vi "Pack Data and Write to Inline.vi"(8 "Error In":errorcluster, 10 "Injection Event Data Cluster":T1 {"Shots"."Results"."Off-Stage Avg Current" format="%#.6g"; "Shots"."Results"."Total Voltage Pulses" format="%#.6g"; "Shots"."Results"."Off-Stage Min Current" format="%#.6g"; "Shots"."Results"."Off-Stage Max Current" format="%#.6g"}, 11 "Async Parameters":T4={"Name"="", "Rate.Hz"=0, "Injectors.Count"=0, "Injector.Timeout"=0.0, "Injector.Timer"=[], "Injector.Info"=[], "Events.Count"=[], "Event.Parameters"={"Shots"=0, "Shot.InitialVoltage"=0.0, "Shot.Stages"=0, "Stages"=[{"Stage.Dwell.Level"=0.0, "PullIn.Type"=enum."Pull In Transition Dwells", "PullIn.Level"=0.0, "Transition.Type"=enum."Stage Transition Voltage Level", "Transition.Level"=0.0}]}, "DMA.Ref"=refnum, "Waveform.Refs"=[], "Waveform.Sessions"=[], "Waveform.Enable"=refnum, "FPGA.Status"=refnum, "Search.Data"=refnum, "Results.Data"=refnum, "Results.Values"=[], "Results.Selections"=[]}) -> (0 "Error out":errorcluster, 3 "Async Parameters out":T4={"Name"="", "Rate.Hz"=0, "Injectors.Count"=0, "Injector.Timeout"=0.0, "Injector.Timer"=[], "Injector.Info"=[], "Events.Count"=[], "Event.Parameters"={"Shots"=0, "Shot.InitialVoltage"=0.0, "Shot.Stages"=0, "Stages"=[{"Stage.Dwell.Level"=0.0, "PullIn.Type"=enum."Pull In Transition Dwells", "PullIn.Level"=0.0, "Transition.Type"=enum."Stage Transition Voltage Level", "Transition.Level"=0.0}]}, "DMA.Ref"=refnum, "Waveform.Refs"=[], "Waveform.Sessions"=[], "Waveform.Enable"=refnum, "FPGA.Status"=refnum, "Search.Data"=refnum, "Results.Data"=refnum, "Results.Values"=[], "Results.Selections"=[]})   [LabVIEW 2015, in "Fuel Injection Addon Engine.lvlib"]
uses:
  Fuel Injection Addon Engine.lvlib
  Types/Async Parameters.ctl
  Shared/Types/Injector info.ctl
  Shared/Types/Shot.Parameters.ctl
  Shared/Types/Stage.Parameters.ctl
  Shared/Types/Stage.PullIn.Types.ctl
  Shared/Types/Stage.Transition.Types.ctl
  <vilib>/NI Veristand/Custom Device API/Waveform Data Reference.ctl
  <vilib>/NI VeriStand/Custom Device Waveform API/Single Waveform Write (DBL)/Single Waveform Write (DBL).lvclass
  <vilib>/NI/NIVS Inline Async API/_Data Access Engine/Data Access Engine/Types/Read.DVR.ctl
  <vilib>/NI/NIVS Inline Async API/_Data Access Engine/Access Type Classes/Read/Read.lvclass
  <vilib>/NI/NIVS Inline Async API/_Data Access Engine/Data Access Engine/Types/Write.DVR.ctl
  <vilib>/NI/NIVS Inline Async API/_Data Access Engine/Access Type Classes/Write/Write.lvclass
  Shared/Types/Analysis.Channels.Select.ctl
  Types/Injector Event Data Cluster.ctl
  RT Analysis/Controls/Shot Information Control.ctl
  Types/Boost Stage Current Measurements Cluster Control.ctl
  <vilib>/NI/NIVS Inline Async API/_Data Access Engine/Access Type Classes/Write/Write.lvclass/Write.ctl
  <vilib>/NI/NIVS Inline Async API/_Data Access Engine/Data Access Engine/Methods/Write.Data.vi
  <vilib>/NI/NIVS Inline Async API/_Data Access Engine/Access Type Classes/Write/Write.ProcessData.vi
  <vilib>/NI/NIVS Inline Async API/_Data Access Engine/Data Access Engine/Data Access Engine.lvclass
  Shared/Fuel Injection Addon Shared.lvlib
  <vilib>/NI VeriStand/Custom Device API/Custom Device API.lvlib
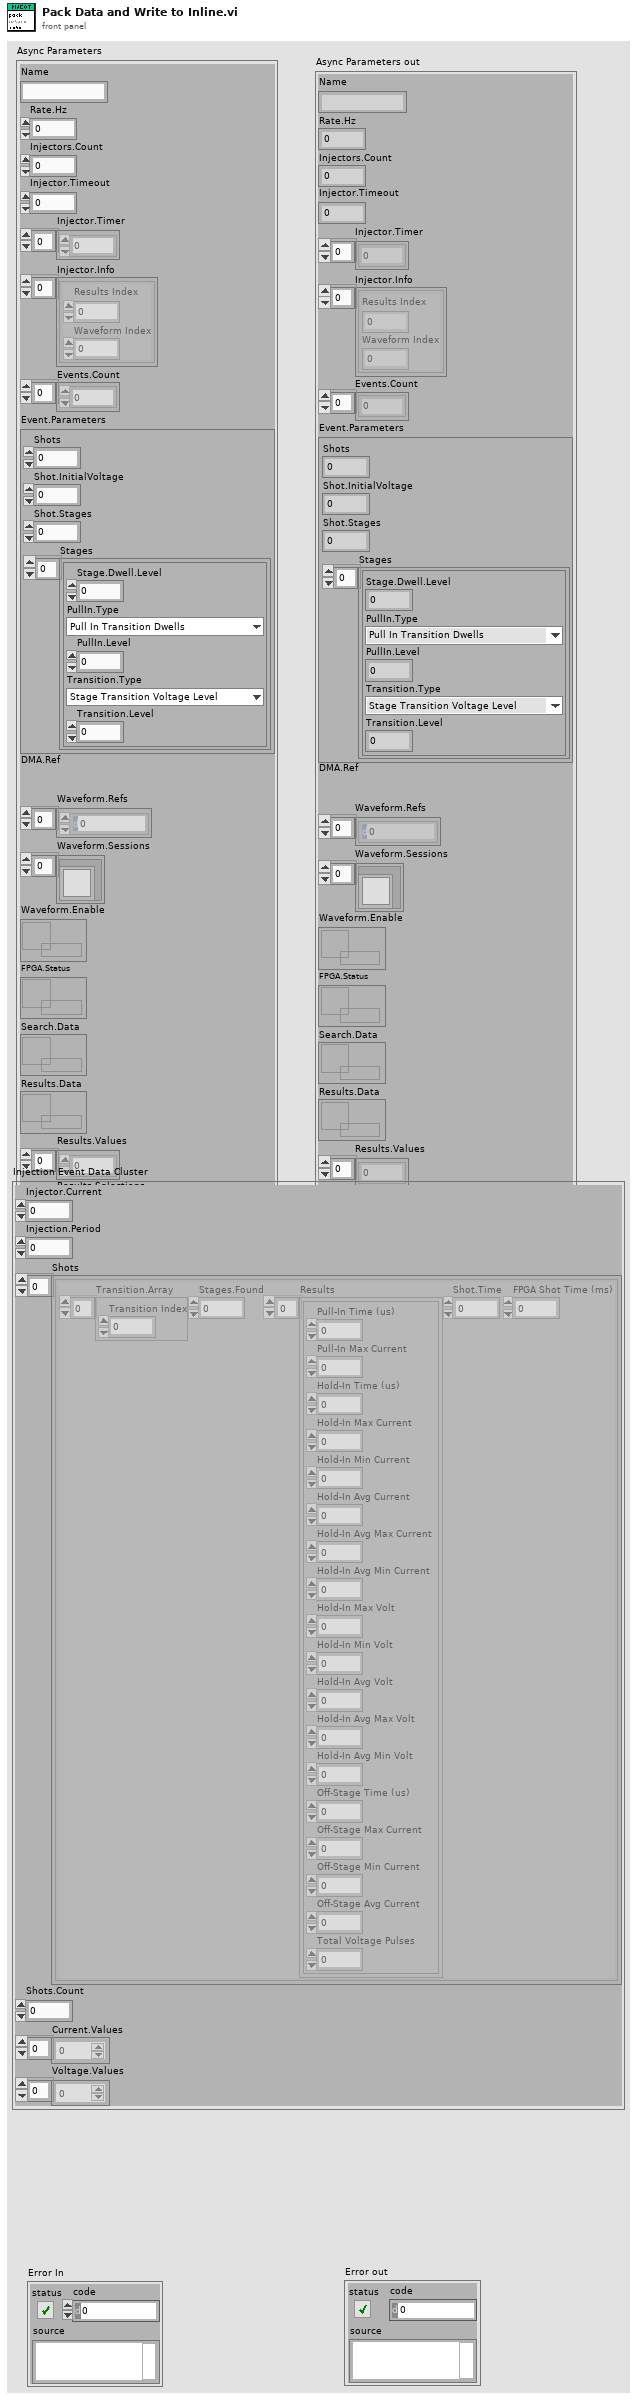
[diagram p1: front panel]
types:
  T1 = typedef "Fuel Injection Addon Engine.lvlib/Injector Event Data Cluster.ctl" = cluster{"Injector.Current":i16, "Injection.Period":dbl, "Shots":T2[], "Shots.Count":i32, "Current.Values":dbl[], "Voltage.Values":dbl[]}
  T2 = typedef "Fuel Injection Addon Engine.lvlib/Shot Information Control.ctl" = cluster{"Transition.Array":i32[], "Stages.Found":u16, "Results":T3[], "Shot.Time":dbl, "FPGA Shot Time (ms)":dbl}
  T3 = typedef "Fuel Injection Addon Engine.lvlib/Boost Stage Current Measurements Cluster Control.ctl" = cluster{"Pull-In Time (us)":dbl, "Pull-In Max Current":dbl, "Hold-In Time (us)":dbl, "Hold-In Max Current":dbl, "Hold-In Min Current":dbl, "Hold-In Avg Current":dbl, "Hold-In Avg Max Current":dbl, "Hold-In Avg Min Current":dbl, "Hold-In Max Volt":dbl, "Hold-In Min Volt":dbl, "Hold-In Avg Volt":dbl, "Hold-In Avg Max Volt":dbl, "Hold-In Avg Min Volt":dbl, "Off-Stage Time (us)":dbl, "Off-Stage Max Current":dbl, "Off-Stage Min Current":dbl, "Off-Stage Avg Current":dbl, "Total Voltage Pulses":dbl}
  T4 = typedef "Fuel Injection Addon Engine.lvlib/Async Parameters.ctl" = cluster{"Name":string, "Rate.Hz":u32, "Injectors.Count":u8, "Injector.Timeout":dbl, "Injector.Timer":u32[], "Injector.Info":T5[], "Events.Count":u64[], "Event.Parameters":T6, "DMA.Ref":refnum<k20>, "Waveform.Refs":T10[], "Waveform.Sessions":refnum<class "Single Waveform Write (DBL).lvclass">[], "Waveform.Enable":T11, "FPGA.Status":T12, "Search.Data":T11, "Results.Data":T12, "Results.Values":dbl[], "Results.Selections":T13[]}
  T5 = typedef "Fuel Injection Addon Shared.lvlib/Injector info.ctl" = cluster{"Results Index":i32, "Waveform Index":i32}
  T6 = typedef "Fuel Injection Addon Shared.lvlib/Shot.Parameters.ctl" = cluster{"Shots":u32, "Shot.InitialVoltage":dbl, "Shot.Stages":u32, "Stages":T7[]}
  T7 = typedef "Fuel Injection Addon Shared.lvlib/Stage.Parameters.ctl" = cluster{"Stage.Dwell.Level":dbl, "PullIn.Type":T8, "PullIn.Level":dbl, "Transition.Type":T9, "Transition.Level":dbl}
  T8 = typedef "Fuel Injection Addon Shared.lvlib/Stage.PullIn.Types.ctl" = enum8{"Pull In Transition Dwells", "Pull In Transition Current Drop"}
  T9 = typedef "Fuel Injection Addon Shared.lvlib/Stage.Transition.Types.ctl" = enum8{"Stage Transition Dwell Time", "Stage Transition Voltage Level", "Stage Transition Current Drop"}
  T10 = typedef "Custom Device API.lvlib/Waveform Data Reference.ctl" = i32
  T11 = typedef "Data Access Engine.lvlib/Data Access Engine.lvclass/Read.DVR.ctl" = refnum<data-value>
  T12 = typedef "Data Access Engine.lvlib/Data Access Engine.lvclass/Write.DVR.ctl" = refnum<data-value>
  T13 = typedef "Fuel Injection Addon Shared.lvlib/Analysis.Channels.Select.ctl" = cluster{"Pull In Time":bool, "Pull In Max Current":bool, "Hold In Time":bool, "Hold In Max Current":bool, "Hold In Min Current":bool, "Hold In Avg Current":bool, "Hold In Avg Max Current":bool, "Hold In Avg Min Current":bool, "Hold In Max Volt":bool, "Hold In Min Volt":bool, "Hold In Avg Volt":bool, "Hold In Avg Max Volt":bool, "Hold In Avg Min Volt":bool, "Off Time":bool, "Off-Stage Max Current":bool, "Off-Stage Min Current":bool, "Off-Stage Avg Current":bool, "Total Voltage Pulses":bool}
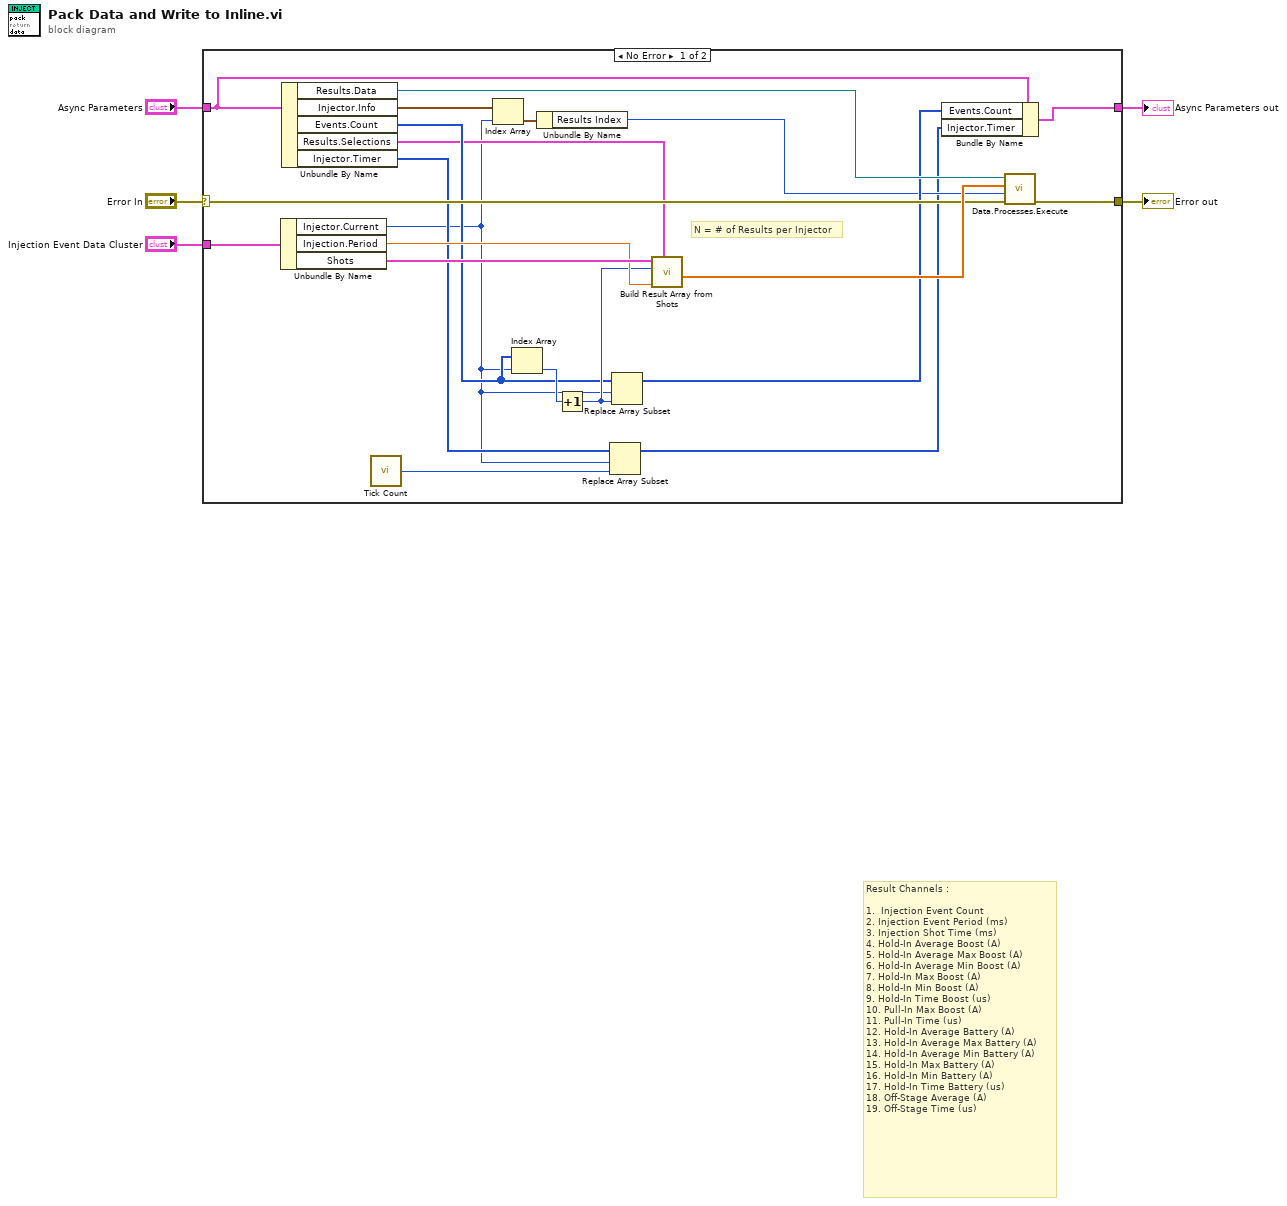
[diagram p0: block diagram]
diagram:
  # "Result Channels :\n\n1.  Injection Event Count\n2. Injection Event Period (ms)\n3. Injection Shot Time (ms)\n4. Hold-In Average Boost (A)\n5. Hold-In Average Max Boost (A)\n6. Hold-In Average Min Boost (A)\n7. Hold-In Max Boost (A)\n8. Hold-In Min Boost (A)\n9. Hold-In Time Boost (us)\n10. Pull-In Max Boost (A)\n11. Pull-In Time (us)\n12. Hold-In Average Battery (A)\n13. Hold-In Average Max Battery (A)\n14. Hold-In Average Min Battery (A)\n15. Hold-In Max Battery (A)\n16. Hold-In Min Battery (A)\n17. Hold-In Time Battery (us)\n18. Off-Stage Average (A)\n19. Off-Stage Time (us)"
  n1 = case shown="No Error" "Error In" {
    selector: "Error In" -> [w20 w28]
    tunnel: [w26 w28] -> w3
    tunnel: "Async Parameters" -> [w16 w27]
    tunnel: [w15 w27] -> w2
    tunnel: "Injection Event Data Cluster" -> [w24 _]
    frame No Error {
      # "N = # of Results per Injector"
      n2 = Unbundle By Name(w24) -> ("Injector.Current"=w7:i16, "Injection.Period"=w22:dbl, "Shots"=w23:T2[])
      n3 = Unbundle By Name(w16) -> ("Results.Data"=w25:T12, "Injector.Info"=w13:T5[], "Events.Count"=w17:u64[], "Results.Selections"=w10:T13[], "Injector.Timer"=w9:u32[])
      n4 = call "Tick Count"() -> ("Tick Count(mSec)"=w6:u32)
      n5 = Index Array(array=w13, index=w7) -> (element=w12:T5)
      n6 = Index Array(array=w17, index=w7) -> (element=w19:u64)
      n7 = Unbundle By Name(w12) -> ("Results Index"=w11:i32)
      n8 = Increment(x=w19) -> (x+1=w18:u64)
      n9 = Replace Array Subset(array=w9, new element=w6, index=w7) -> (w8:u32[])
      n10 = Replace Array Subset(array=w17, new element=w18, index=w7) -> (w14:u64[])
      n11 = call "Build Result Array from Shots.vi"("Analysis Selections"=w10, "Injection Event Dwell Period (ms)"=w22, "Injection Event Count"=w18, "Shot Info Array"=w23) -> ("Result Array"=w21:dbl[])  [unwired: 7 in]
      n12 = Bundle By Name(cluster=w16, "Events.Count"=w14, "Injector.Timer"=w8) -> (w15:T4)
      n13 = call-poly <vilib>:"Data.Processes.Execute.vi"("error in (no error)"=w20, "Offset"=w11, "Values"=w21, "Ref"=w25) -> ("error out"=w26:errorcluster)  [unwired: 7 in]
    }
    frame Error {
    }
  }
  "Error out" <- w3
  "Async Parameters out" <- w2
